vi "DepthSense NewFrame Callback.vi"(4 "User Parameter":variant, 6 "Control Ref":refnum<k24>, 7 "Event Common Data":T1) -> ()   [LabVIEW 2011]
uses:
  C:/Users/Behavior Room/Desktop/Kinect Mouse/DepthSense/FunctionPointerProxy/FunctionPointerProxy/bin/Release/FunctionPointerProxy.dll
  FunctionPointerProxy/FunctionPointerProxy/bin/Release/FunctionPointerProxy.dll
  <vilib>/Utility/importsl/GetValueByPointer/datatype.ctl
  IT WORKS SO SUCK IT/DepthSense Global Status.vi
  <vilib>/Utility/importsl/GetValueByPointer/GetValueByPointer.xnode
  Program Files (x86)/National Instruments/LabVIEW 2011/resource/lvimptsl.dll
  <userlib>/libOptrima-2-3/libOptrima-2-3.lvlib
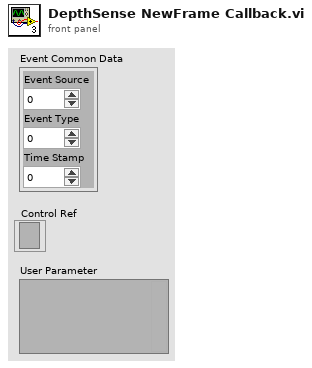
[diagram p1: front panel]
types:
  T1 = cluster{"Event Source":i32, "Event Type":u32, "Time Stamp":u32}
  T2 = typedef "Image Type" = u32
  T3 = cluster{"Camera Version":string, "Image Height":i32, "Image Width":i32, "Minimum Framerate":i32, "Maximum Framerate":i32, "Framerate":i32, "Close Mode":bool, "Denoising":bool, "Leakage Algorithm":bool, "Anti-Aliasing":bool, "Camera Status":i32, "API Version":string, "Light Intensity":i32, "Confidence Threshold":u16, "Range":sgl}
  T4 = typedef "IMAQ Image.ctl" = refnum<image>
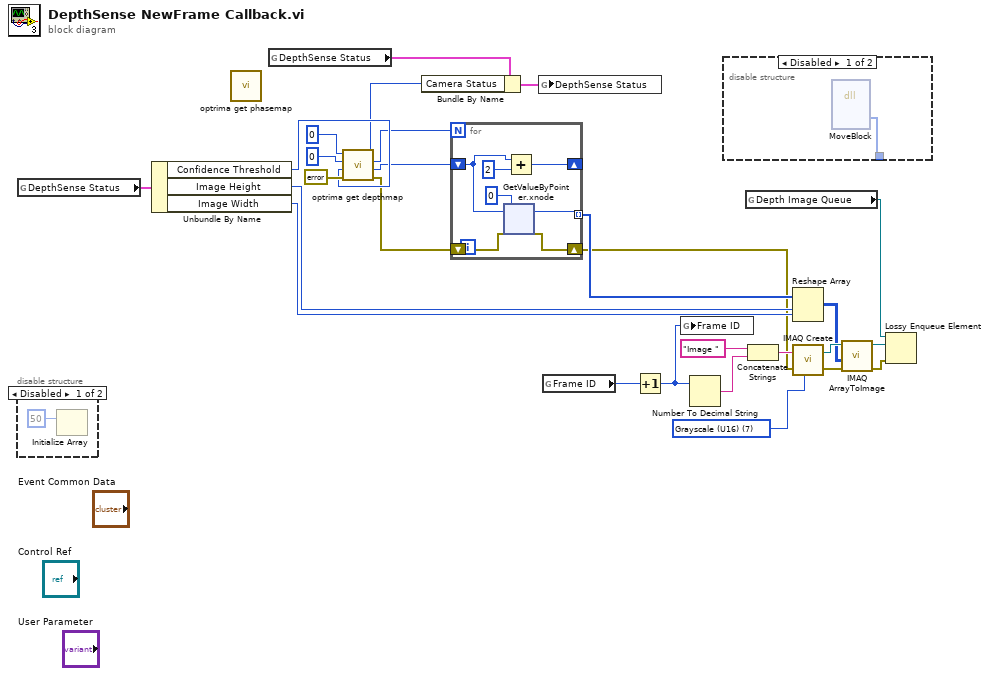
[diagram p0: block diagram]
diagram:
  w16 = T2 7 items=["Grayscale (U8)", "Grayscale (I16)", "Grayscale (SGL)", "Complex (CSG)", "RGB (U32)", "HSL (U32)", "RGB (U64)", "Grayscale (U16)"] ("Image Type")
  n1 = global read "DepthSense Global Status.vi" "DepthSense Status"() -> (w27:T3)
  n2 = disable-structure shown="Disabled" {
    frame Disabled {
      n3 = Initialize Array(i16 50 ("element")) -> ()  [unwired: 1 in, 1 out]
    }
    frame Enabled {
    }
  }
  n4 = Unbundle By Name(w27) -> ("Confidence Threshold"=w7:u16, "Image Height"=w22:i32, "Image Width"=w21:i32)
  n5 = call <userlib>:"optrima get phasemap.vi"() -> ()  [unwired: 8 in, 4 out]
  n6 = global read "DepthSense Global Status.vi" "DepthSense Status"() -> (w25:T3)
  n7 = call <userlib>:"optrima get depthmap.vi"("error in (no error)"=errorcluster {"status"=FALSE, "code"=0, "source"=""}, "confidenceTH"=w7, "length"=u32 0, "p_depthmap"=0 ("p_phase_map")) -> ("error out"=w4:errorcluster, "p_depthmap out"=w5:i32, "length out"=w2:u32, "function return"=w1:u32)  [unwired: 4 in]
  n8 = Bundle By Name(cluster=w25, "Camera Status"=w1) -> (w26:T3)
  n9 = for {
    N: w2 -> [_]
    tunnel: [w35] -> w10 mode=indexing
    shift-right: [w32] -> _
    shift-left: w5 -> [w31]
    shift-right: [w29] -> w3
    shift-left: w4 -> [w30]
    n10 = xnode "GetValueByPointer.xnode"("Pointer"=w31, "InputType"=0 ("p_phase_map"), "ErrorIn"=w30) -> ("Output"=w35:i32, "ErrorOut"=w29:errorcluster)  [unwired: 1 in]
    n11 = Add(x=w31, y=2) -> (x+y=w32:i32)
  }
  n12 = global write "DepthSense Global Status.vi" "DepthSense Status"(w26) -> ()
  n13 = global read "DepthSense Global Status.vi" "Frame ID"() -> (w23:i32)
  n14 = Increment(x=w23) -> (x+1=w20:i32)
  n15 = global write "DepthSense Global Status.vi" "Frame ID"(w20) -> ()
  n16 = Number To Decimal String(number=w20) -> (decimal integer string=w19:string)  [unwired: 1 in]
  n17 = disable-structure shown="Disabled" {
    disable-tunnel: [w44 _] -> _
    frame Disabled {
      n18 = dll-call lib="LabVIEW" fn="MoveBlock"() -> ("dst"=w44:i32[])  [unwired: 9 in, 2 out]
    }
    frame Enabled {
    }
  }
  n19 = global read "DepthSense Global Status.vi" "Depth Image Queue"() -> (w24:refnum<queue>)
  n20 = Concatenate Strings("Image " ("Image Name"), w19) -> (w17:string)
  n21 = Reshape Array(w10, w22, w21) -> (w11:i32[][])
  n22 = call "IMAQ Create"("Image Name"=w17, "Image Type"=w16, "error in (no error)"=w3) -> ("New Image"=w14:T4, "error out"=w15:errorcluster)  [unwired: 2 in]
  n23 = call "IMAQ ArrayToImage"("error in (no error)"=w15, "Image Pixels (I16)"=w11, "Image"=w14) -> ("error out"=w12:errorcluster, "Image Out"=w13:T4)  [unwired: 7 in]
  n24 = Lossy Enqueue Element(queue=w24, element=w13, error in (no error)=w12) -> ()  [unwired: 4 out]
